vi "g_ChipData.vi"() -> ()   [LabVIEW 2014]
panel:
  out "Success Alignment":bool[][](array[boolean]) caption="Occupied"
  out "Testresults":bool[][](array[boolean]) caption="Occupied"
  out "Active Y":dbl
  out "Active X":dbl
  out "Tested":bool[][](array[boolean]) caption="Occupied"
  out "Alignment Processed":bool[][](array[boolean]) caption="Occupied"
  out "Occupied":bool[][](array[boolean])
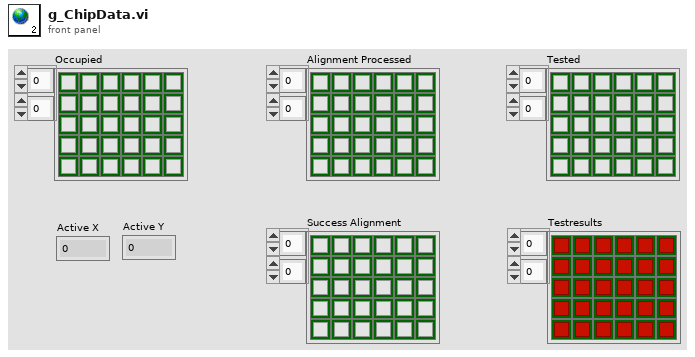
[diagram p1: front panel]
diagram:
